vi "Pitch Angle Compensation_2.vi"(9 "Pitch Calib":T1={"Array"=[[80.0, 1.0, 1.0, 1.0, 1.0, 1.0, 1.0, 1.0, 1.0], [70.0, 0.875, 0.0, 0.0, 0.0, 0.0, 0.0, 0.0, 0.0], [60.0, 0.75, 0.0, 0.0, 0.0, 0.0, 0.0, 0.0, 0.0], [50.0, 0.625, 0.0, 0.0, 0.0, 0.0, 0.0, 0.0, 0.0], [40.0, 0.5, 0.0, 0.0, 0.0, 0.0, 0.0, 0.0, 0.0], [30.0, 0.375, 0.0, 0.0, 0.0, 0.0, 0.0, 0.0, 0.0], [20.0, 0.25, 0.0, 0.0, 0.0, 0.0, 0.0, 0.0, 0.0], [10.0, 0.125, 0.0, 0.0, 0.0, 0.0, 0.0, 0.0, 0.0], [0.0, 0.0, 0.0, 0.0, 0.0, 0.0, 0.0, 0.0, 0.0], [-10.0, -0.125, 0.0, 0.0, 0.0, 0.0, 0.0, 0.0, 0.0], [-20.0, -0.25, 0.0, 0.0, 0.0, 0.0, 0.0, 0.0, 0.0], [-30.0, -0.375, 0.0, 0.0, 0.0, 0.0, 0.0, 0.0, 0.0], [-40.0, -0.5, 0.0, 0.0, 0.0, 0.0, 0.0, 0.0, 0.0], [-50.0, -0.625, 0.0, 0.0, 0.0, 0.0, 0.0, 0.0, 0.0], [-60.0, -0.75, 0.0, 0.0, 0.0, 0.0, 0.0, 0.0, 0.0], [-70.0, -0.875, 0.0, 0.0, 0.0, 0.0, 0.0, 0.0, 0.0], [-80.0, -1.0, 0.0, 0.0, 0.0, 0.0, 0.0, 0.0, 0.0]], "Operation"=FALSE}, 11 "Sensor Input":dbl) -> (3 "Pitch Angle":dbl)   [LabVIEW 2017]
uses:
  Pitch Array 1.ctl
  <vilib>/gmath/NI_Gmath.lvlib
panel:
  # "Calibration\nMode"
  # "Operating\nMode"
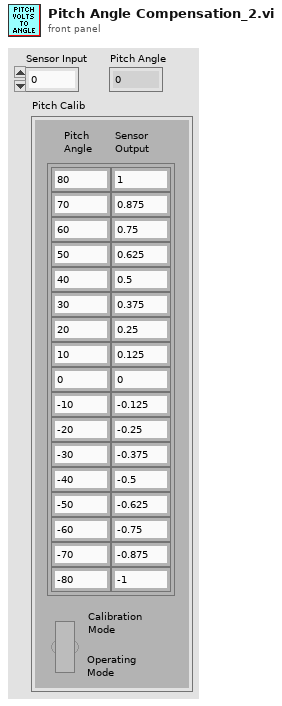
[diagram p1: front panel]
types:
  T1 = typedef "Pitch Array 1.ctl" = cluster{"Array":dbl[][], "Operation":bool}
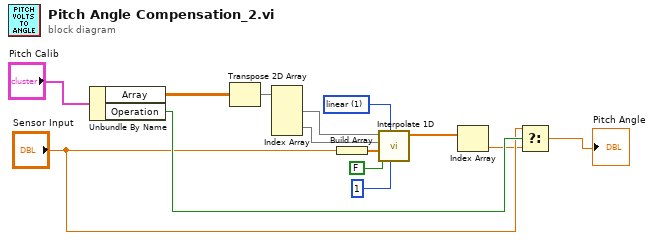
[diagram p0: block diagram]
diagram:
  w12 = 1 items=["nearest", "linear", "spline", "cubic Hermite", "Lagrange"] ("method")
  n1 = Unbundle By Name("Pitch Calib") -> ("Array"=w8:dbl[][], "Operation"=w3:bool)
  n2 = Transpose 2D Array(2D array=w8) -> (transposed array=w7:dbl[][])
  n3 = Index Array(array=w7) -> (element #1=w6:dbl[], element #2=w5:dbl[])  [unwired: 4 in]
  n4 = Build Array("Sensor Input") -> (w11:dbl[])
  n5 = call <vilib>:"Interpolate 1D.vi"("ntimes"=1, "method"=w12, "X is monotonic"=FALSE, "xi"=w11, "X"=w5, "Y"=w6) -> ("yi"=w10:dbl[])  [unwired: 3 in, 2 out]
  n6 = Index Array(array=w10) -> (element=w1:dbl)  [unwired: 1 in]
  n7 = Select(t="Sensor Input", s=w3, f=w1) -> (s? t:f=→"Pitch Angle":dbl)
